vi "Ui_Manette_Monitor.vi"() -> ()   [LabVIEW 2018]
uses:
  SwerveDrive.ctl
  <vilib>/Utility/inputDevices.llb/joystickAcquire.vi
  <vilib>/Utility/inputDevices.llb/closeJoystick.vi
panel:
  out "SwerveDrive":T1
  out "direction info":T2
  out "Y Rotation":dbl(graph)
  out "X Rotation":dbl(graph)
  out "Z axis":dbl(graph)
  out "Y Axis":dbl(graph)
  out "X Axis":dbl(graph)
  in  "stop":bool
  out "axis info":T3
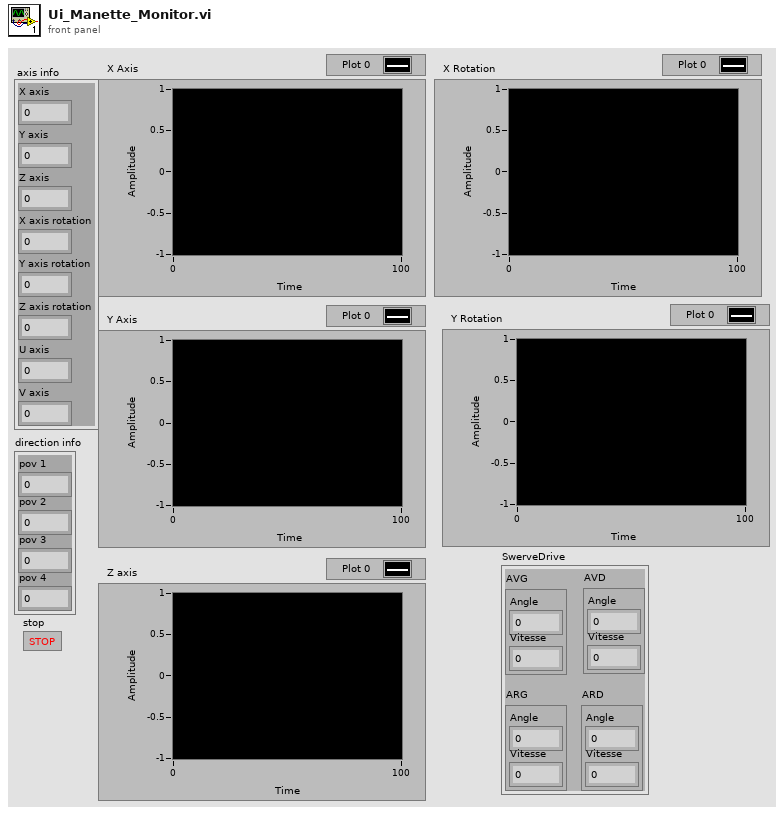
[diagram p1: front panel]
types:
  T1 = typedef "SwerveDrive.ctl" = cluster{"AVD":cluster{"Angle":dbl, "Vitesse":dbl}, "AVG":cluster{"Angle":dbl, "Vitesse":dbl}, "ARG":cluster{"Angle":dbl, "Vitesse":dbl}, "ARD":cluster{"Angle":dbl, "Vitesse":dbl}}
  T2 = cluster{"pov 1":i32, "pov 2":i32, "pov 3":i32, "pov 4":i32}
  T3 = cluster{"X axis":i32, "Y axis":i32, "Z axis":i32, "X axis rotation":i32, "Y axis rotation":i32, "Z axis rotation":i32, "U axis":i32, "V axis":i32}
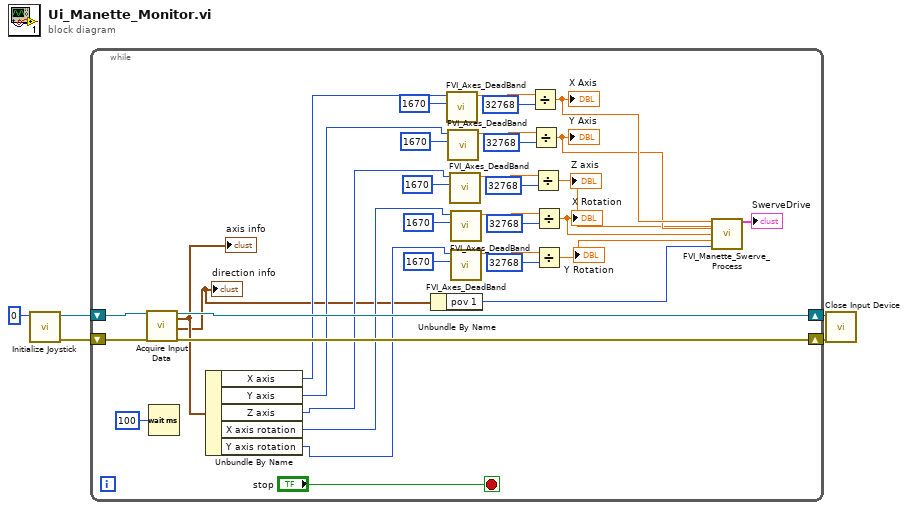
[diagram p0: block diagram]
diagram:
  n1 = call <vilib>:"Initialize Joystick.vi"("device index"=0) -> ("error out"=w3:errorcluster, "device ID"=w5:refnum<k1>)  [unwired: 9 in]
  n2 = while {
    shift-right: [w37] -> w1
    shift-left: w5 -> [w40]
    shift-right: [w38] -> w2
    shift-left: w3 -> [w39]
    stop <- "stop" stop-if-true
    n3 = call-poly <vilib>:"Acquire Input Data.vi"("device ID"=w40, "error in (no error)"=w39) -> ("device ID"=w37:refnum<k1>, "axis info"=w34:T3, "direction info"=w13:T2, "error out"=w38:errorcluster)  [unwired: 13 in, 1 out]
    "axis info" <- w34
    "direction info" <- w13
    n4 = Wait (ms)(milliseconds to wait=u32 100) -> ()  [unwired: 1 out]
    n5 = Unbundle By Name(w34) -> ("X axis"=w32:i32, "Y axis"=w26:i32, "Z axis"=w16:i32, "X axis rotation"=w15:i32, "Y axis rotation"=w14:i32)
    n6 = Unbundle By Name(w13) -> ("pov 1"=w8:i32)
    n7 = call "FVI_Axes_DeadBand.vi"("deadband Value"=1670 ("x"), "X axis in"=w32) -> ("X axis out"=w31:dbl)  [unwired: 8 in, 1 out]
    n8 = call "FVI_Axes_DeadBand.vi"("deadband Value"=1670 ("x"), "X axis in"=w26) -> ("X axis out"=w28:dbl)  [unwired: 8 in, 1 out]
    n9 = call "FVI_Axes_DeadBand.vi"("deadband Value"=1670 ("x"), "X axis in"=w16) -> ("X axis out"=w24:dbl)  [unwired: 8 in, 1 out]
    n10 = call "FVI_Axes_DeadBand.vi"("deadband Value"=1670 ("x"), "X axis in"=w15) -> ("X axis out"=w21:dbl)  [unwired: 8 in, 1 out]
    n11 = call "FVI_Axes_DeadBand.vi"("deadband Value"=1670 ("x"), "X axis in"=w14) -> ("X axis out"=w18:dbl)  [unwired: 8 in, 1 out]
    n12 = Divide(x=w31, y=32768) -> (x/y=w12:dbl)
    "X Axis" <- w12
    n13 = Divide(x=w28, y=32768) -> (x/y=w11:dbl)
    "Y Axis" <- w11
    n14 = Divide(x=w24, y=32768) -> (x/y=w7:dbl)
    "Z axis" <- w7
    n15 = Divide(x=w21, y=32768) -> (x/y=w10:dbl)
    "X Rotation" <- w10
    n16 = Divide(x=w18, y=32768) -> (x/y=w9:dbl)
    "Y Rotation" <- w9
    n17 = call "FVI_Manette_Swerve_Process.vi"("Axe L X"=w12, "Ltrigger"=w7, "Axe L Y"=w11, "Axe R X"=w10, "Axe R Y"=w9, "POV"=w8) -> ("SwerveDrive"=→"SwerveDrive":T1)  [unwired: 9 in]
  }
  n18 = call-poly <vilib>:"Close Input Device.vi"("error in (no error)"=w2, "device ID"=w1) -> ()  [unwired: 8 in, 1 out]
